vi "set_offset.vi"(8 "error in (no error)":errorcluster, 10 "offset":dbl[unit][](array[numeric]), 11 "FPGAWrapperMH120124FrameScan_PXI7813R in":refnum<class "FPGAWrapperMH120124FrameScan_PXI7813R.lvclass">) -> (0 "error out":errorcluster, 3 "FPGAWrapperMH120124FrameScan_PXI7813R out":refnum<class "FPGAWrapperMH120124FrameScan_PXI7813R.lvclass">)   [LabVIEW 2010, in "FPGAWrapperMH120124FrameScan_PXI7813R.lvclass"]
uses:
  FPGAWrapperMH120124FrameScan_PXI7813R.lvclass
  FPGAWrapperMH120124FrameScan_PXI7813R.lvclass/FPGAWrapperMH120124FrameScan_PXI7813R.ctl
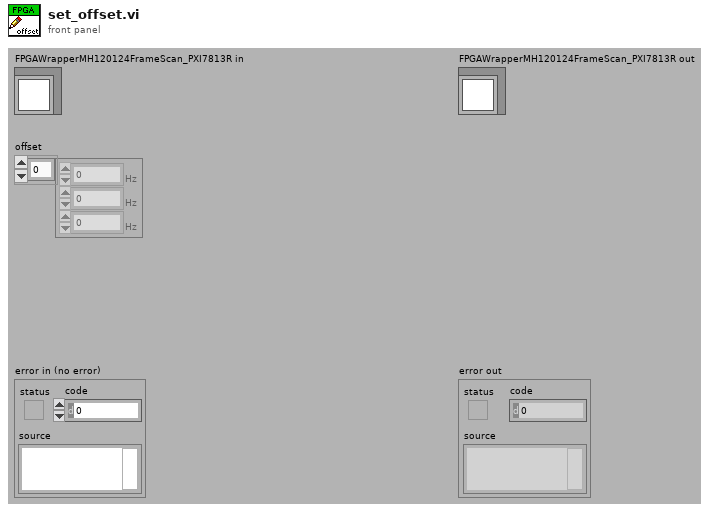
[diagram p1: front panel]
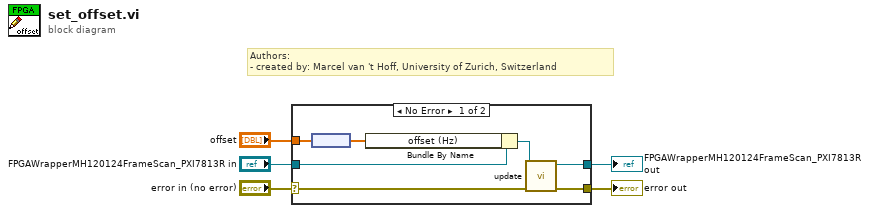
[diagram p0: block diagram]
diagram:
  # "Authors: \n- created by: Marcel van 't Hoff, University of Zurich, Switzerland"
  n1 = case shown="No Error" "error in (no error)" {
    selector: "error in (no error)" -> [w9 w13]
    tunnel: [w8 w13] -> w4
    tunnel: [w6 w14] -> w2
    tunnel: "FPGAWrapperMH120124FrameScan_PXI7813R in" -> [w12 w14]
    tunnel: "offset" -> [w11 _]
    frame No Error {
      n2 = node(w11) -> (w10:dbl[])
      n3 = Bundle By Name(cluster=w12, "offset (Hz)"=w10) -> (w7:refnum<class "FPGAWrapperMH120124FrameScan_PXI7813R.lvclass">)
      n4 = call-dynamic "update.vi"("error in (no error)"=w9, "FPGAWrapperMH120124FrameScan_PXI7813R in"=w7) -> ("error out"=w8:errorcluster, "FPGAWrapperMH120124FrameScan_PXI7813R out"=w6:refnum<class "FPGAWrapperMH120124FrameScan_PXI7813R.lvclass">)  [unwired: 8 in]
    }
    frame Error {
    }
  }
  "error out" <- w4
  "FPGAWrapperMH120124FrameScan_PXI7813R out" <- w2
